vi "Get Encodings.vi"(8 "error in (no error)":errorcluster, 11 "Encoding in":refnum<class "CConfig Automatic Encoding.lvclass">) -> (0 "error out":errorcluster, 3 "Encoding out":refnum<class "CConfig Automatic Encoding.lvclass">, 4 "Encodings":refnum<class "CConfig Encoding.lvclass">[](array[class]))   [LabVIEW 2013, in "CConfig Automatic Encoding.lvclass"]
doc: "Copyright 2018, Carya Automatisering, Wiebe Walstra."
uses:
  CConfig Automatic Encoding.lvclass
  CConfig Encoding.lvclass
  CConfig Automatic Encoding.lvclass/CConfig Automatic Encoding.ctl
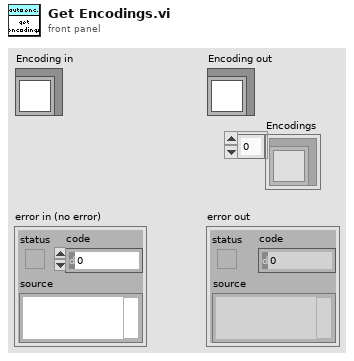
[diagram p1: front panel]
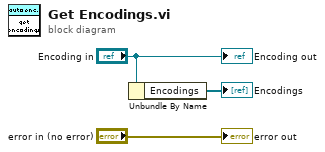
[diagram p0: block diagram]
diagram:
  n1 = Unbundle By Name("Encoding in") -> ("Encodings"=→"Encodings":refnum<class "CConfig Encoding.lvclass">[])
  "error out" <- "error in (no error)"
  "Encoding out" <- "Encoding in"
